vi "tcp发送-main.vi"(0 "对方网络地址":string="127.0.0.1", 5 "原文件路径（使用对话框）":path=path "C:/Users/Administrator.2W964MZOGI5HE3B/Desktop/labview图片/105256rhad11pc5553vz5e.png") -> (4 "运行指示灯":bool=TRUE, 6 "已传百分比":string)   [LabVIEW 2016, in "TCP发送文件.lvlib"]
panel:
  out "数值":i32
  in  "分帧数(兆)":i64=2
  out "已发帧数":i32
  in  "分一包（兆）":i64=40
  out "侦数":i32
  out "在发第几次":i32
  out "共发送次数":string
  out "网络灯":bool
  in  "停止":bool
  out "错误输出 2":errorcluster caption="错误输出"
  out "错误输出":errorcluster
  out "文件名称":string
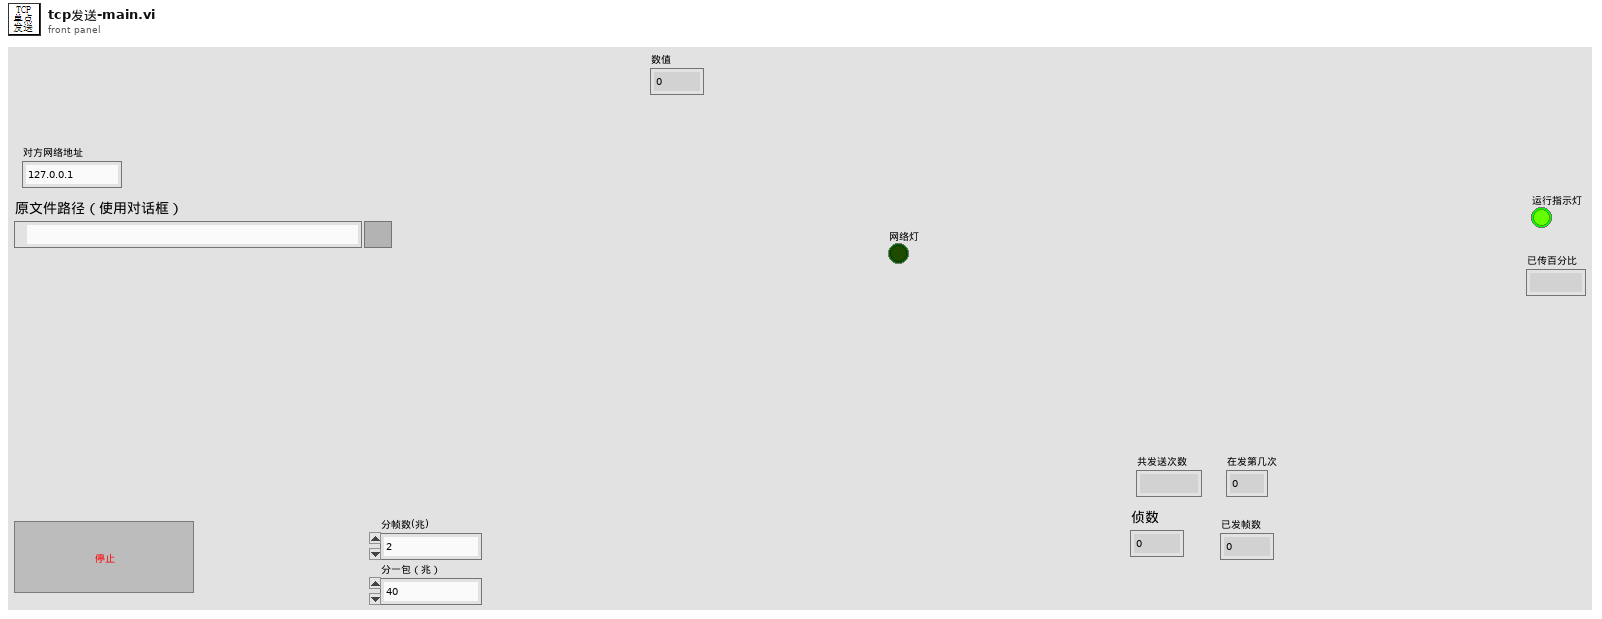
[diagram p1: front panel]
types:
  T1 = enum16{"open", "replace", "create", "open or create", "replace or create", "replace or create with confirmation"}
  T2 = cluster{"网络灯":bool, "发送中":bool, "已发送百分比":string, "发送成功次数":dbl}
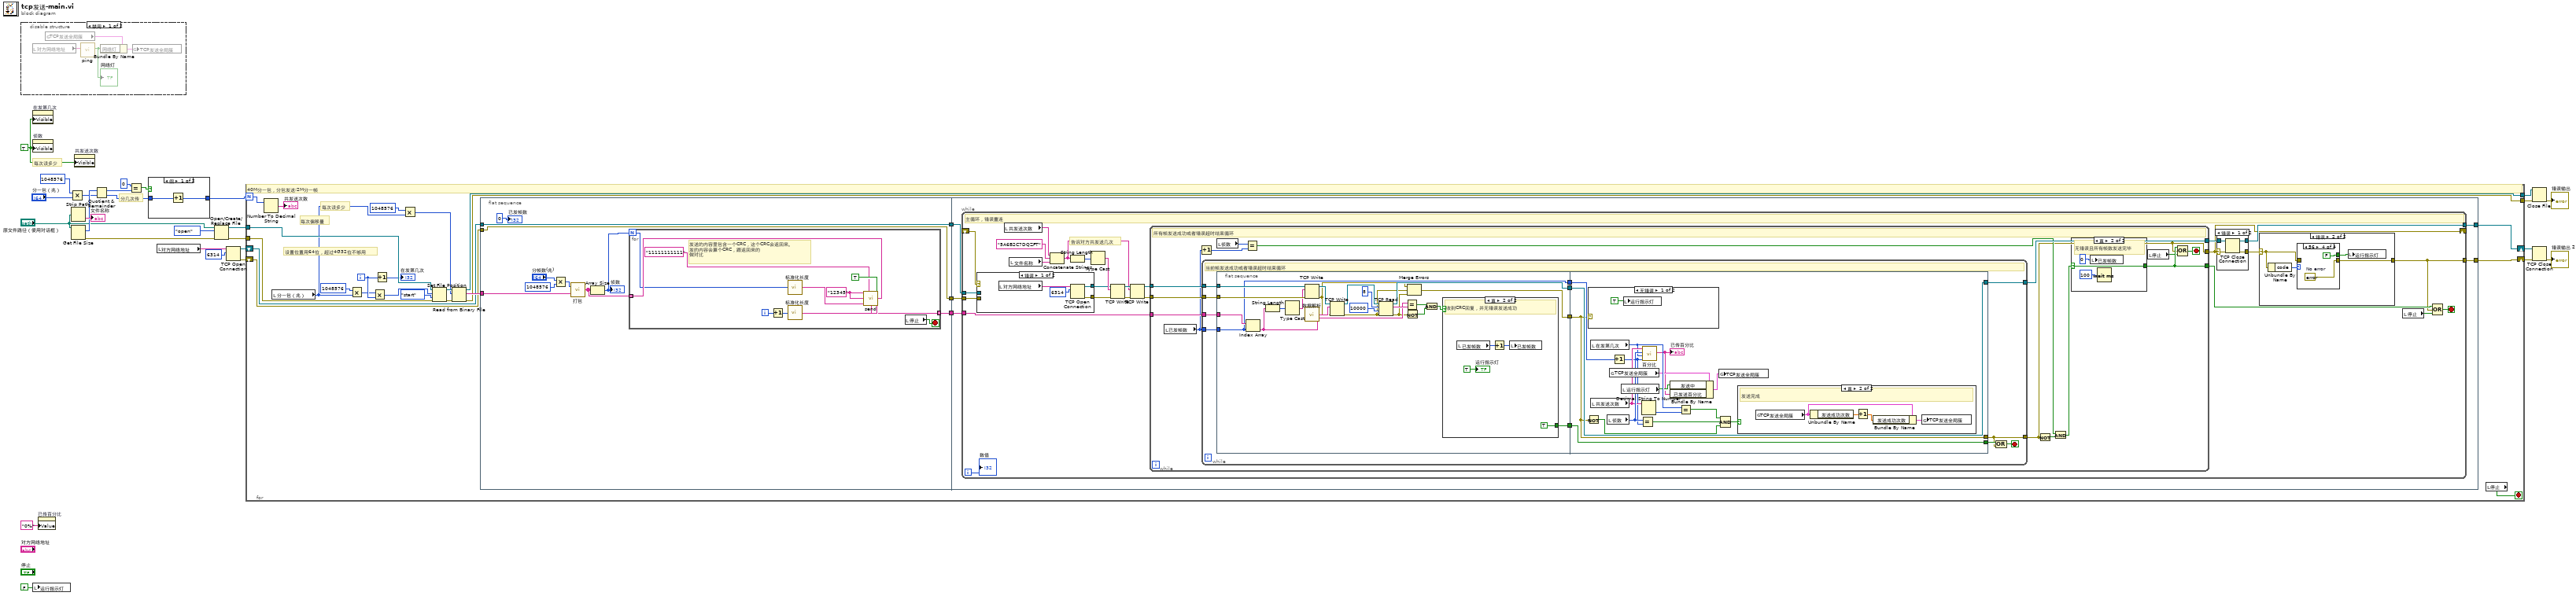
[diagram p0: block diagram]
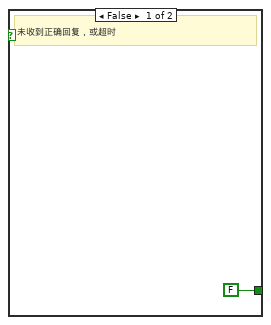
[diagram p7: hidden frame]
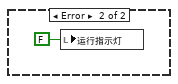
[diagram p8: hidden frame]
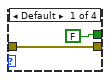
[diagram p11: hidden frame]
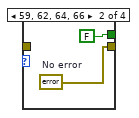
[diagram p12: hidden frame]
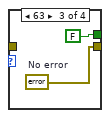
[diagram p13: hidden frame]
diagram:
  w11 = TRUE ("可见")
  # "分几次传"
  # "每次读多少"
  n1 = disable-structure shown="禁用" {
    frame Disabled {
      n2 = local read "对方网络地址"() -> (w32:string)
      n3 = global read "全局变量1.vi" "TCP发送全局簇"() -> (w30:T2)
      n4 = call "ping.vi"("IP"=w32) -> ("ping结果"=w29:bool)  [unwired: 10 in]
      "网络灯" <- w29
      n5 = Bundle By Name(cluster=w30, "网络灯"=w29) -> (w31:T2)
      n6 = global write "全局变量1.vi" "TCP发送全局簇"(w31) -> ()
    }
    frame Enabled {
    }
  }
  n7 = property on="在发第几次" class="DigNum (严格)"("Visible"=w11) -> ()  [unwired: 2 in, 2 out]
  n8 = property on="侦数" class="DigNum (严格)"("Visible"=w11) -> ()  [unwired: 2 in, 2 out]
  n9 = local write "运行指示灯"(FALSE ("运行指示灯")) -> ()
  n10 = property on="已传百分比" class="Str"("Value"="0%" ("已传百分比")) -> ()  [unwired: 2 in, 2 out]
  n11 = Multiply(x=i64 1048576 ("y"), y="分一包（兆）") -> (x*y=w2:i64)
  n12 = Strip Path(path="原文件路径（使用对话框）") -> (name=→"文件名称":string)  [unwired: 1 out]
  n13 = Get File Size(file="原文件路径（使用对话框）") -> (size (in bytes)=w8:i64, 0:w9:errorcluster)  [unwired: 1 in, 1 out]
  n14 = property on="共发送次数" class="Str"("Visible"=w11) -> ()  [unwired: 2 in, 2 out]
  n15 = Quotient & Remainder(x=w8, y=w2) -> (x-y*floor(x/y)=w25:i64, floor(x/y)=w21:i64)
  n16 = Equal?(x=0, y=w25) -> (x = y?=w23:bool)
  n17 = case shown="假" w23 {
    tunnel: [w33 w35] -> w22
    tunnel: w21 -> [w34 w35]
    frame False {
      n18 = Increment(x=w34) -> (x+1=w33:i64)
    }
    frame True {
    }
  }
  n19 = local read "对方网络地址"() -> (w10:string)
  n20 = Open/Create/Replace File(file path (use dialog)="原文件路径（使用对话框）", error in=w9, operation (0:open)=T1."open" ("操作(0:open)")) -> (refnum out=w6:refnum<file>, error out=w5:errorcluster)  [unwired: 3 in, 1 out]
  n21 = TCP Open Connection(address=w10, remote port or service name=u16 6314 ("远程端口或服务名称")) -> (connection ID=w13:refnum<k5>, error out=w12:errorcluster)  [unwired: 3 in]
  n22 = for {
    N: w22 -> [w42]
    tunnel: w5 -> [w57]
    tunnel: w6 -> [w56]
    tunnel: [w52] -> w19
    tunnel: [w51] -> w20
    shift-right: [w46] -> w15
    shift-left: w13 -> [w45]
    shift-right: [w47] -> w16
    shift-left: w12 -> [w44]
    i -> [w50]
    stop <- w36 stop-if-true
    # "设置位置用64位，超过4G32位不够用"
    # "每次读多少"
    # "每次偏移量"
    # "40M分一包，分包发送;2M分一帧"
    n23 = Number To Decimal String(number=w42) -> (decimal integer string=→"共发送次数":string)  [unwired: 1 in]
    n24 = local read "分一包（兆）"() -> (w38:i64)
    n25 = Multiply(x=i64 1048576 ("偏移量（字节）（0）"), y=w38) -> (x*y=w40:i64)
    n26 = Multiply(x=w40, y=w50) -> (x*y=w58:i64)
    n27 = Increment(x=w50) -> (x+1=→"在发第几次":i32)
    n28 = Multiply(x=1048576 ("总数(1)"), y=w38) -> (x*y=w37:i64)
    n29 = Set File Position(offset (in bytes) (0)=w58, refnum=w56, from (0:start)=enum16{"start", "end", "current"}."start" ("自（0:起始）"), error in=w57) -> (refnum out=w60:refnum<file>, error out=w61:errorcluster)
    n30 = Read from Binary File(8:w61, 10:w37, 11:w60) -> (0:w52:errorcluster, 2:w55:string, 3:w51:refnum<file>)  [unwired: 3 in, 1 out]
    n31 = flat-sequence {
      tunnel: w55 -> [w66]
      tunnel: [w69] -> w53
      tunnel: [w68] -> w49
      tunnel: w45 -> [w68]
      tunnel: [w67] -> w48
      tunnel: w44 -> [w67]
      tunnel: w53 -> [w87]
      tunnel: w49 -> [w86]
      tunnel: w48 -> [w85]
      tunnel: [w84] -> w47
      tunnel: [w83] -> w46
      frame #0 {
        n32 = Multiply(x="分帧数(兆)", y=i64 1048576) -> (x*y=w65:i64)
        n33 = call "打包.vi"("总内容"=w66, "分包大小"=w65) -> ("分包数组"=w64:string[])
        n34 = Array Size(array=w64) -> (size(s)=w71:i32)
        "侦数" <- w71
        n35 = for {
          N: w71 -> [w77]
          tunnel: w64 -> [w82] mode=indexing
          tunnel: [w75] -> w69 mode=indexing
          i -> [w81]
          stop <- w72 stop-if-true
          w74 = "12345" ("内容说明（文件名）")
          # "发送的内容里包含一个CRC，这个CRC会返回来。\n发的内容会算个CRC，跟返回来的\n做对比"
          n36 = Increment(x=w81) -> (x+1=w76:i32)
          n37 = call "标准化长度.vi"("原长度"=w77) -> ("标准化长度"=w80:string)
          n38 = call "标准化长度.vi"("原长度"=w76) -> ("标准化长度"=w79:string)
          n39 = call "send.vi"("内容标识"=w74, "时标"="11111111111", "发送"=TRUE, "内容说明（文件名）"=w74, "帧内容"=w82, "帧数"=w80, "帧号"=w79) -> ("连接的字符串"=w75:string)  [unwired: 6 in, 2 out]
          n40 = local read "停止"() -> (w72:bool)
        }
        "已发帧数" <- 0 ("数值")
      }
      frame #1 {
        n41 = while {
          tunnel: w87 -> [w98]
          tunnel: w86 -> [w97]
          tunnel: w85 -> [w96]
          tunnel: [w95] -> w84
          tunnel: [w94] -> w83
          shift-right: [w93] -> _
          shift-left: _ -> [w92]
          i -> [w88]
          stop <- w110 stop-if-true
          # "告诉对方共发送几次"
          # "主循环，错误重连"
          n42 = case shown="错误" w92 {
            tunnel: [w122 w124] -> w91
            tunnel: w97 -> [_ w124]
            tunnel: [w121 w123] -> w90
            tunnel: w96 -> [_ w123]
            frame Error {
              n43 = local read "对方网络地址"() -> (w120:string)
              n44 = TCP Open Connection(address=w120, remote port or service name=u16 6314 ("远程端口或服务名称")) -> (connection ID=w122:refnum<k5>, error out=w121:errorcluster)  [unwired: 3 in]
            }
            frame No Error {
            }
          }
          n45 = local read "共发送次数"() -> (w101:string)
          n46 = local read "文件名称"() -> (w102:string)
          n47 = Concatenate Strings(w101, "5A6B2C7DQZFT" ("字符串"), w102) -> (w99:string)
          n48 = String Length(string=w99) -> (length=w108:i32)
          n49 = Type Cast(x=w108) -> (*(type *) &x=w107:string)  [unwired: 1 out]
          n50 = TCP Write(connection ID=w91, data in=w107, error in (no error)=w90) -> (connection ID out=w105:refnum<k5>, error out=w106:errorcluster)  [unwired: 2 out]
          n51 = TCP Write(connection ID=w105, data in=w99, error in (no error)=w106) -> (connection ID out=w104:refnum<k5>, error out=w103:errorcluster)  [unwired: 2 out]
          n52 = while {
            tunnel: w104 -> [w138]
            tunnel: w103 -> [w136]
            tunnel: [w127] -> w93
            tunnel: [w134] -> w112
            tunnel: [w132] -> w109
            tunnel: w98 -> [w133]
            stop <- w137 stop-if-true
            # "所有帧发送成功或者错误超时结束循环"
            n53 = local read "已发帧数"() -> (w131:i32)
            n54 = Increment(x=w131) -> (x+1=w130:i32)
            n55 = while {
              tunnel: w131 -> [w153]
              tunnel: w133 -> [w151]
              tunnel: w138 -> [w154]
              tunnel: [w150] -> w134
              tunnel: w136 -> [w152]
              tunnel: [w148] -> w127
              stop <- w147 stop-if-true
              # "当前帧发送成功或者错误超时结束循环"
              n56 = flat-sequence {
                tunnel: w154 -> [w175]
                tunnel: w153 -> [w162]
                tunnel: w152 -> [w174]
                tunnel: w151 -> [w171]
                tunnel: [w169] -> w146
                tunnel: [w168] -> w145
                tunnel: [w155] -> w144
                tunnel: [w162] -> w143
                tunnel: [w187] -> w148
                tunnel: [w198] -> w149
                tunnel: [w199] -> w150
                tunnel: w146 -> [w199]
                tunnel: w145 -> [w198]
                tunnel: w144 -> [w187]
                tunnel: w143 -> [w190]
                frame #0 {
                  n57 = Index Array(array=w171, index=w162) -> (element=w167:string)
                  n58 = String Length(string=w167) -> (length=w176:i32)
                  n59 = Type Cast(x=w176) -> (*(type *) &x=w170:string)  [unwired: 1 out]
                  n60 = TCP Write(connection ID=w175, data in=w170, error in (no error)=w174) -> (connection ID out=w177:refnum<k5>, error out=w157:errorcluster)  [unwired: 2 out]
                  n61 = call "数据解析.vi"("data in"=w167) -> ("data out"=w166:string, "CRC"=w164:string)  [unwired: 4 in, 9 out]
                  n62 = TCP Write(connection ID=w177, data in=w166, error in (no error)=w157) -> (connection ID out=w173:refnum<k5>, error out=w156:errorcluster)  [unwired: 2 out]
                  n63 = TCP Read(connection ID=w173, bytes to read=8 ("读取的字节"), error in (no error)=w156, 9:10000 ("超时毫秒(25000)")) -> (connection ID out=w169:refnum<k5>, data out=w165:string, error out=w158:errorcluster)  [unwired: 1 in]
                  n64 = Equal?(x=w164, y=w165) -> (x = y?=w161:bool)
                  n65 = Not(x=w158) -> (.not. x?=w160:bool)
                  n66 = Merge Errors(w157, w156, w158) -> (w155:errorcluster)
                  n67 = And(x=w161, y=w160) -> (x .and. y?=w159:bool)
                  n68 = case shown="真" w159 {
                    tunnel: [FALSE TRUE] -> w168
                    frame False {
                      # "未收到正确回复，或超时"
                    }
                    frame True {
                      # "收到CRC回复，并无错误发送成功"
                      n69 = local read "已发帧数"() -> (w181:i32)
                      n70 = Increment(x=w181) -> (x+1=w182:i32)
                      n71 = local write "已发帧数"(w182) -> ()
                      "运行指示灯" <- TRUE
                    }
                  }
                }
                frame #1 {
                  n72 = Not(x=w187) -> (.not. x?=w188:bool)
                  n73 = case shown="无错误" w187 {
                    frame No Error {
                      n74 = local write "运行指示灯"(TRUE ("运行指示灯")) -> ()
                    }
                    frame Error {
                      n75 = local write "运行指示灯"(FALSE ("运行指示灯")) -> ()
                    }
                  }
                  n76 = local read "在发第几次"() -> (w194:i32)
                  n77 = local read "共发送次数"() -> (w196:string)
                  n78 = local read "侦数"() -> (w197:i32)
                  n79 = global read "全局变量1.vi" "TCP发送全局簇"() -> (w184:T2)
                  n80 = Increment(x=w190) -> (x+1=w189:i32)
                  n81 = local read "运行指示灯"() -> (w186:bool)
                  n82 = Equal?(x=w197, y=w189) -> (x = y?=w192:bool)
                  n83 = Decimal String To Number(string=w196) -> (number=w195:i32)  [unwired: 2 in, 1 out]
                  n84 = call "百分比.vi"("已发帧数 2"=w189, "发第几次"=w194, "帧数"=w197, "共发送次数"=w196) -> ("已传百分比"=w183:string)  [unwired: 7 in]
                  "已传百分比" <- w183
                  n85 = Bundle By Name(cluster=w184, "发送中"=w186, "已发送百分比"=w183) -> (w185:T2)
                  n86 = Equal?(x=w194, y=w195) -> (x = y?=w193:bool)
                  n87 = global write "全局变量1.vi" "TCP发送全局簇"(w185) -> ()
                  n88 = Compound Arithmetic op=AND(w193, w192, w188) -> (w191:bool)
                  n89 = case shown="真" w191 {
                    frame False {
                    }
                    frame True {
                      # "发送完成"
                      n90 = global read "全局变量1.vi" "TCP发送全局簇"() -> (w202:T2)
                      n91 = Unbundle By Name(w202) -> ("发送成功次数"=w203:dbl)
                      n92 = Increment(x=w203) -> (x+1=w204:dbl)
                      n93 = Bundle By Name(cluster=w202, "发送成功次数"=w204) -> (w205:T2)
                      n94 = global write "全局变量1.vi" "TCP发送全局簇"(w205) -> ()
                    }
                  }
                }
              }
              n95 = Compound Arithmetic op=OR(w149, w148) -> (w147:bool)
            }
            n96 = local read "侦数"() -> (w135:i32)
            n97 = Equal?(x=w135, y=w130) -> (x = y?=w129:bool)
            n98 = Not(x=w127) -> (.not. x?=w126:bool)
            n99 = Compound Arithmetic op=AND(w129, w126) -> (w128:bool)
            n100 = case shown="真" w128 {
              selector: w128 -> [w139 w141]
              tunnel: [w139 w141] -> w132
              frame False {
              }
              frame True {
                # "无错误且所有帧数发送完毕"
                n101 = local write "已发帧数"(0 ("已发帧数")) -> ()
                n102 = Wait (ms)(milliseconds to wait=u32 100 ("等待时间（毫秒）")) -> ()  [unwired: 1 out]
              }
            }
            n103 = local read "停止"() -> (w125:bool)
            n104 = Compound Arithmetic op=OR(w132, w127, w125) -> (w137:bool)
          }
          n105 = case shown="错误" w93 {
            selector: w93 -> [w113 w117]
            tunnel: w112 -> [w116 w118]
            tunnel: [w115 w117] -> w111
            tunnel: [w114 w118] -> w94
            frame Error {
              n106 = TCP Close Connection(connection ID=w116, error in (no error)=w113) -> (connection ID out=w114:refnum<k5>, error out=w115:errorcluster)  [unwired: 1 in]
            }
            frame No Error {
            }
          }
          n107 = case shown="错误" w111 {
            selector: w111 -> [w206 w209]
            tunnel: [w206 w208] -> w95
            frame No Error {
            }
            frame Error {
              n108 = Unbundle By Name(w209) -> ("code"=w210:i32)
              n109 = case shown="56" w210 {
                tunnel: w209 -> [w212 _ _ _]
                tunnel: [w212 w214 w216 w218] -> w208
                tunnel: [FALSE FALSE FALSE FALSE] -> w207
                frame Default {
                }
                frame 59, 62, 64, 66 {
                  w214 = errorcluster {"status"=FALSE, "code"=0, "source"=""}  # No error
                }
                frame 63 {
                  w216 = errorcluster {"status"=FALSE, "code"=0, "source"=""}  # No error
                }
                frame 56 {
                  w218 = errorcluster {"status"=FALSE, "code"=0, "source"=""}  # No error
                }
              }
              n110 = local write "运行指示灯"(w207) -> ()
            }
          }
          n111 = local read "停止"() -> (w89:bool)
          n112 = Compound Arithmetic op=OR(w109, w95, w89) -> (w110:bool)
          "数值" <- w88
        }
      }
    }
    n113 = local read "停止"() -> (w36:bool)
  }
  n114 = Close File(refnum=w20, error in=w19) -> (error out=→"错误输出":errorcluster)  [unwired: 1 out]
  n115 = TCP Close Connection(connection ID=w15, error in (no error)=w16) -> (error out=→"错误输出 2":errorcluster)  [unwired: 1 in, 1 out]
